vi "Read First Write.vi"(8 "error in (no error)":errorcluster, 11 "TDMS-Actor in":refnum<class "TDMS-Actor.lvclass">=refnum) -> (0 "error out":errorcluster, 2 "First Write":bool, 3 "TDMS-Actor out":refnum<class "TDMS-Actor.lvclass">)   [LabVIEW 2016, in "BNT_TDMS.lvlib" / "TDMS-Actor.lvclass"]
uses:
  TDMS-Actor.lvclass
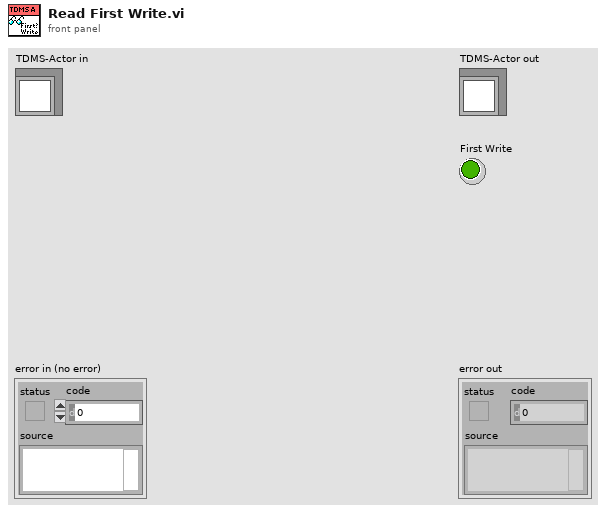
[diagram p1: front panel]
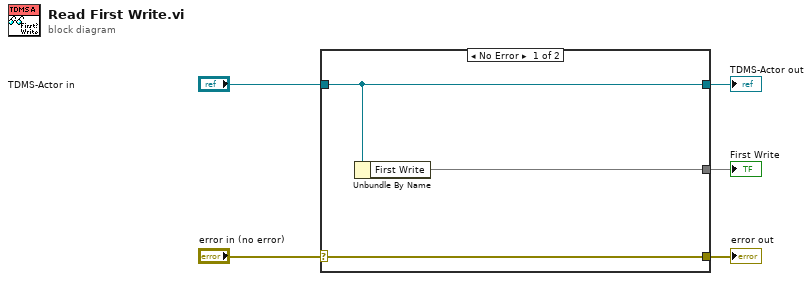
[diagram p0: block diagram]
diagram:
  n1 = case shown="No Error" "error in (no error)" {
    selector: "error in (no error)" -> [w8 w9]
    tunnel: [w8 w9] -> w4
    tunnel: [w7 w10] -> w2
    tunnel: "TDMS-Actor in" -> [w7 w10]
    tunnel: [w6 _] -> w1
    frame No Error {
      n2 = Unbundle By Name(w7) -> ("First Write"=w6)
    }
    frame Error {
    }
  }
  "error out" <- w4
  "TDMS-Actor out" <- w2
  "First Write" <- w1
